vi "Write SG Pin.vi"(8 "error in (no error)":errorcluster, 10 "SG Pin":string, 11 "ET_Delay_Sweep in":refnum<class "ET_Delay_Sweep.lvclass">) -> (0 "error out":errorcluster, 3 "ET_Delay_Sweep out":refnum<class "ET_Delay_Sweep.lvclass">)   [LabVIEW 2018, in "SeqAuto Evaluations.lvlib" / "ET_Delay_Sweep.lvclass"]
uses:
  ET_Delay_Sweep.lvclass
  ET_Delay_Sweep.lvclass/ET_Delay_Sweep.ctl
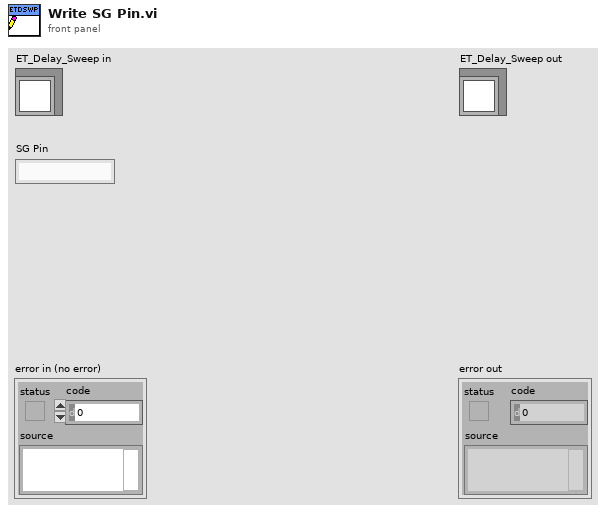
[diagram p1: front panel]
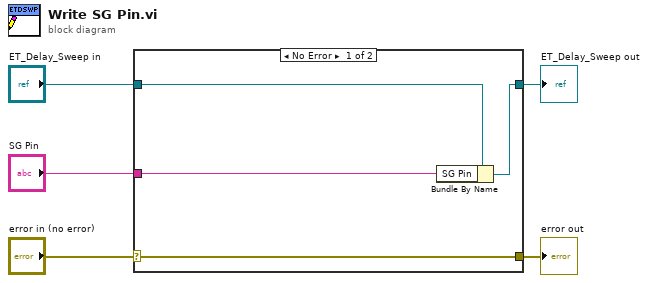
[diagram p0: block diagram]
diagram:
  n1 = case shown="No Error" "error in (no error)" {
    selector: "error in (no error)" -> [w9 w10]
    tunnel: [w9 w10] -> w4
    tunnel: [w7 w11] -> w2
    tunnel: "ET_Delay_Sweep in" -> [w8 w11]
    tunnel: "SG Pin" -> [w6 _]
    frame No Error {
      n2 = Bundle By Name(cluster=w8, "SG Pin"=w6) -> (w7:refnum<class "ET_Delay_Sweep.lvclass">)
    }
    frame Error {
    }
  }
  "error out" <- w4
  "ET_Delay_Sweep out" <- w2
